vi "Get Object.vi"(8 "error in":errorcluster, 9 "Sub-Index":i16=-1, 10 "Index":u16 format="%04x", 11 "reference in":refnum<class "Electronic Datasheet.lvclass">) -> (0 "error out":errorcluster, 1 "OD Entry":refnum<class "OD Entry.lvclass">, 2 "Found?":bool, 3 "reference out":refnum<class "Electronic Datasheet.lvclass">)   [LabVIEW 2024, in "Electronic Datasheet.lvlib" / "Electronic Datasheet.lvclass"]
uses:
  Electronic Datasheet.lvclass
  Core/OD Entry/OD Entry.lvclass
  Core/Sorted Object Dictionary/Sorted Object Dictionary.lvclass
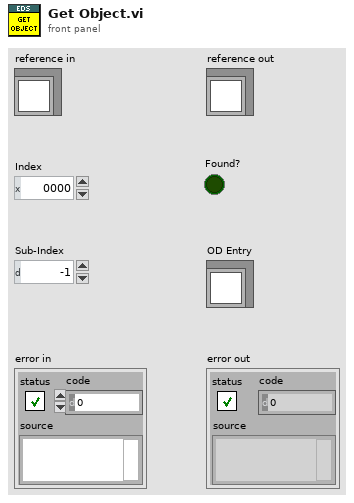
[diagram p1: front panel]
types:
  T1 = typedef "Electronic Datasheet.lvlib/Electronic Datasheet.lvclass/ObjectAttributes.ctl" = cluster{"EDS File Path":path, "Object Dict":refnum<class "Dictionary.lvclass">, "Sorted Object Dict":refnum<class "Sorted Object Dictionary.lvclass">, "Device Info":refnum<class "Device Info.lvclass">, "File Info":refnum<class "File Info.lvclass">}
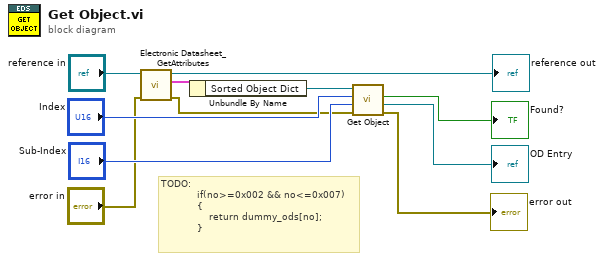
[diagram p0: block diagram]
diagram:
  # "TODO:\n            if(no>=0x002 && no<=0x007)\n            {\n                return dummy_ods[no];\n            }"
  n1 = call "Electronic Datasheet_GetAttributes.vi"("Error In"="error in", "reference in"="reference in") -> ("Error Out"=w4:errorcluster, "Data"=w7:T1, "reference out"=→"reference out":refnum<class "Electronic Datasheet.lvclass">)  [unwired: 6 in, 1 out]
  n2 = Unbundle By Name(w7) -> ("Sorted Object Dict"=w6:refnum<class "Sorted Object Dictionary.lvclass">)
  n3 = call "Get Object.vi"("error in"=w4, "Sub-Index"="Sub-Index", "Index"="Index", "Sorted Object Dictionary in"=w6) -> ("error out"=→"error out":errorcluster, "OD Entry"=→"OD Entry":refnum<class "OD Entry.lvclass">, "Found?"=→"Found?":bool)  [unwired: 4 in, 1 out]
